vi "write_read_subvi_ad7747.vi"(8 "error in (no error)":errorcluster, 9 "Time Delay":bool=TRUE, 10 "command":string="900D80", 11 "Control":refnum<visa-resource-name>) -> (0 "error out":errorcluster, 2 "output":string, 3 "Control out":refnum<visa-resource-name>)   [LabVIEW 2012]
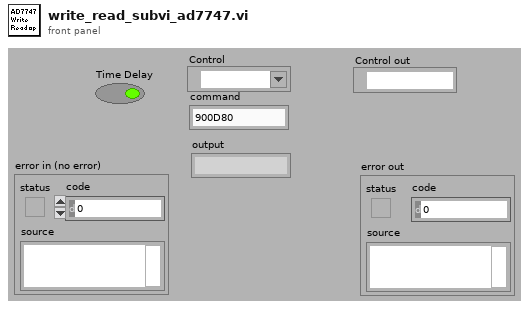
[diagram p1: front panel]
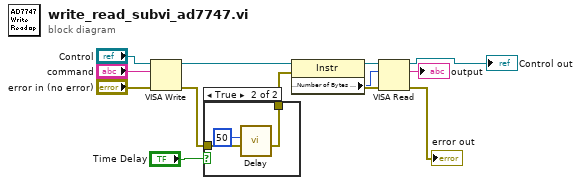
[diagram p0: block diagram]
diagram:
  n1 = VISA Write(VISA resource name="Control", write buffer="command", error in (no error)="error in (no error)") -> (VISA resource name out=w9:refnum<visa-resource-name>, error out=w1:errorcluster)  [unwired: 1 out]
  n2 = case shown="True" "Time Delay" {
    tunnel: w1 -> [w14 w17]
    tunnel: [w14 w16] -> w3
    frame False {
    }
    frame True {
      n3 = call "Delay.vi"("error in (no error)"=w17, "milliseconds to wait"=u32 50) -> ("error out"=w16:errorcluster)  [unwired: 9 in]
    }
  }
  n4 = property class="Instr"(reference=w9, error in=w3) -> (reference out=w11:refnum<visa-resource-name>, error out=w12:errorcluster, "Serial Settings:Number of Bytes at Serial Port"=w4:u32)
  n5 = VISA Read(VISA resource name=w11, byte count=w4, error in (no error)=w12) -> (VISA resource name out=→"Control out":refnum<visa-resource-name>, read buffer=→"output":string, error out=→"error out":errorcluster)  [unwired: 1 out]
